vi "extract_depth_range.vi"(7 "offset":dbl=2.0, 8 "error in (no error)":errorcluster, 9 "size":dbl=2.0, 10 "Image Dst":T1, 11 "Image":T1) -> (0 "error out":errorcluster, 3 "Image Dst Out":T1)   [LabVIEW 2016]
doc: "Extracts ROI from image spanning whole width, with top at y position 'vertical offset' and of height 'vertical size'.\ns"
uses:
  <vilib>/vision/Image Controls.llb/IMAQ Image.ctl
  <vilib>/vision/NI_Vision_Development_Module.lvlib
panel:
  out "co-ordinates":dbl[](array[numeric])
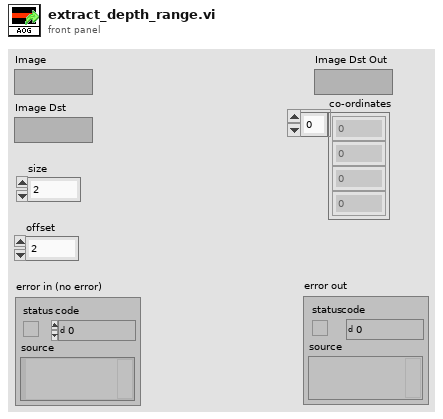
[diagram p1: front panel]
types:
  T1 = typedef "IMAQ Image.ctl" = refnum<image>
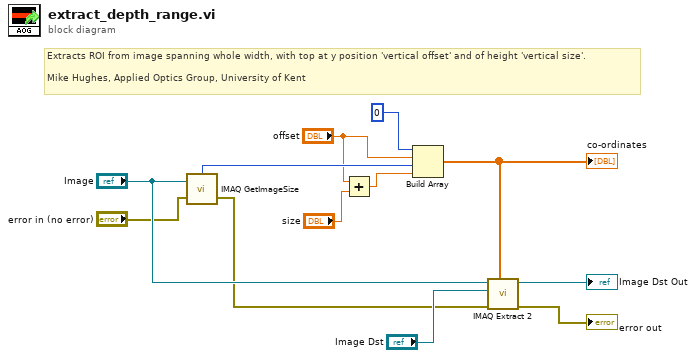
[diagram p0: block diagram]
diagram:
  # "Extracts ROI from image spanning whole width, with top at y position 'vertical offset' and of height 'vertical size'.\n\nMike Hughes, Applied Optics Group, University of Kent"
  n1 = call "IMAQ GetImageSize"("Image"="Image", "error in (no error)"="error in (no error)") -> ("X Resolution"=w6:i32, "error out"=w1:errorcluster)  [unwired: 2 in, 1 out]
  n2 = Add(x="offset", y="size") -> (x+y=w3:dbl)
  n3 = Build Array(0 ("element"), "offset", w6, w3) -> (w11:dbl[])
  "co-ordinates" <- w11
  n4 = call "IMAQ Extract 2"("Optional Rectangle"=w11, "error in (no error)"=w1, "Image Dst"="Image Dst", "Image Src"="Image") -> ("error out"=→"error out":errorcluster, "Image Dst Out"=→"Image Dst Out":T1)  [unwired: 6 in]
